vi "Example - Opening and Editing an Installer.vi"() -> ()   [LabVIEW 2017]
doc: "Demonstrates the use of the Installer Builder API to open, modify, and build an Installer build specification."
uses:
  <vilib>/InstallerBuilder/Classes/Win_Source/AB_Win_Source.lvclass/AB_Win_Source.ctl
  <vilib>/InstallerBuilder/Classes/Win_InstallTime_Executable/Install Time Type.ctl
  <vilib>/InstallerBuilder/Classes/Win_Installer/AB_Win_Installer.lvclass/AB_Win_Installer.ctl
  <vilib>/InstallerBuilder/Classes/Win_Source/Get Name.vi
  <vilib>/InstallerBuilder/Classes/Win_Source/Get Install Path.vi
  <vilib>/InstallerBuilder/Classes/Win_Installer/Get Product Name.vi
  <vilib>/InstallerBuilder/Classes/Win_Installer/Get Product Version.vi
  <vilib>/InstallerBuilder/Classes/Win_Source_File/AB_Win_Source_File.lvclass
  e:/builds/penguin/labview/branches/2017/dev/dist/vi.lib/InstallerBuilder/Classes/Win_Source/AB_Win_Source.lvclass
  <vilib>/InstallerBuilder/Classes/Win_Installer/Get Installed Files.vi
  <vilib>/InstallerBuilder/Classes/Win_Installer/Get System Folder (Desktop).vi
  <vilib>/InstallerBuilder/Classes/Win_Source_File/Set Read Only.vi
  <vilib>/InstallerBuilder/Classes/Win_Installer/Get Registry Hive (Local Machine).vi
  <vilib>/AppBuilder/AB_API_Simple/Build (project reference).vi
  <vilib>/InstallerBuilder/Classes/Win_Installer/AB_Win_Installer.lvclass
  <vilib>/AppBuilder/AB_API_Simple/NI_App_Builder_API.lvlib
  <vilib>/InstallerBuilder/Classes/Win_InstallTime_Executable/AB_Win_InstallTime_Executable.lvclass
panel:
  out "Files included in the installer":string[](array[string])
  # "Overview: Demonstrates the use of the Installer Builder API to open, modify, and build an Installer build specification.\nRequirements: LabVIEW Professional Development System or LabVIEW Application Builder\nInstructions:\n1. Run the VI. The My Installer build specification will be opened, modified, then built programmatically.\n2. A project window will open. Examine the My Installer build specification in the project.\n3. Close the temporary project and delete the temporary project files generated by this example when you are done.\n4. In the Project Explorer window, right-click on the My Installer build specification and choose Explore to navigate to the installer and run it."
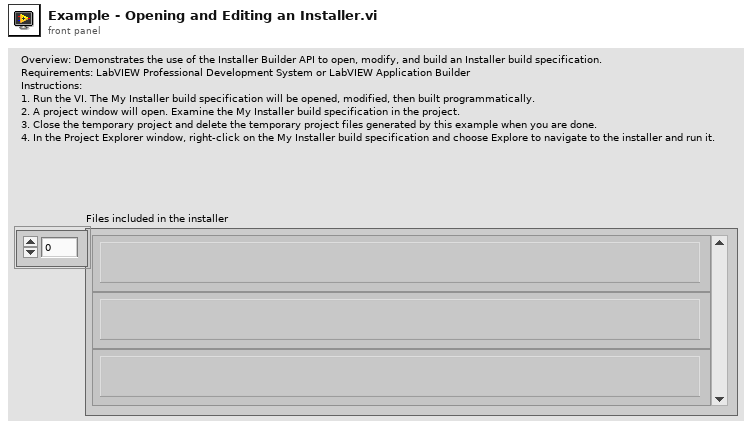
[diagram p1: front panel]
types:
  T1 = typedef "AB_Win_InstallTime_Executable.lvclass/Install Time Type.ctl" = enum16{"After install", "Before uninstall"}
  T2 = typedef "AB_Win_Installer.lvclass/Product Version.ctl" = cluster{"Major":u8, "Minor":u8, "Update":u16}
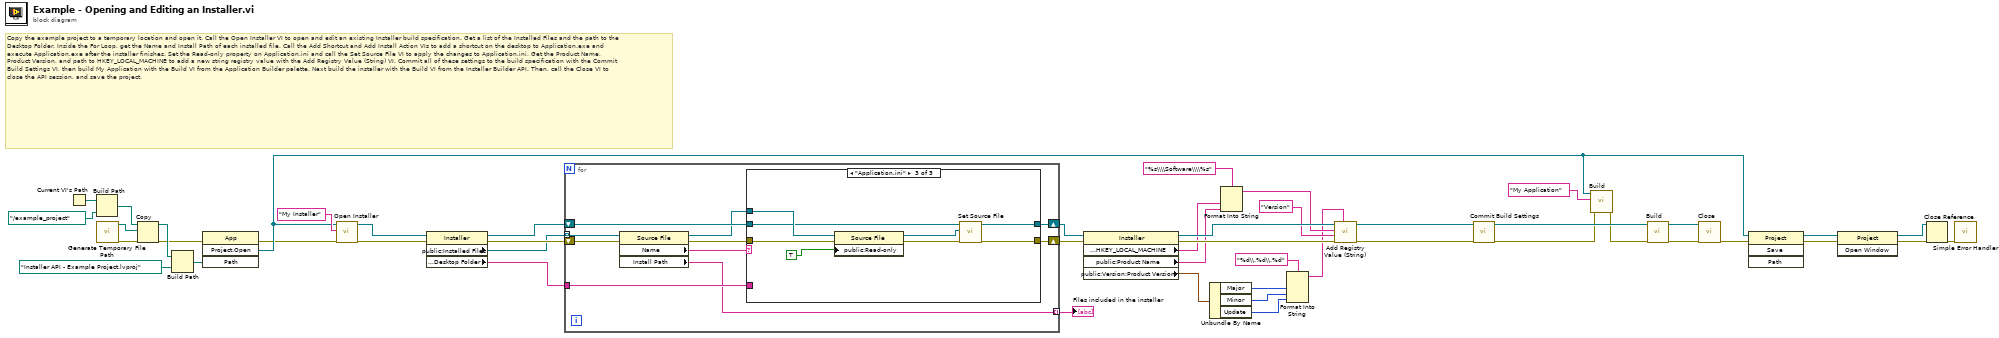
[diagram p0: block diagram]
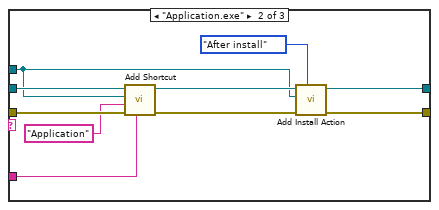
[diagram p3: hidden frame]
diagram:
  # "Copy the example project to a temporary location and open it. Call the Open Installer VI to open and edit an existing Installer build specification. Get a list of the Installed Files and the path to the Desktop Folder. Inside the For Loop, get the Name and Install Path of each installed file. Call the Add Shortcut and Add Install Action VIs to add a shortcut on the desktop to Application.exe and execute Application.exe after the installer finishes. Set the Read-only property on Application.ini and call the Set Source File VI to apply the changes to Application.ini. Get the Product Name, Product Version, and path to HKEY_LOCAL_MACHINE to add a new string registry value with the Add Registry Value (String) VI. Commit all of these settings to the build specification with the Commit Build Settings VI, then build My Application with the Build VI from the Application Builder palette. Next build the installer with the Build VI from the Installer Builder API. Then, call the Close VI to close the API session, and save the project."
  n1 = Current VI's Path() -> (path=w48:path)
  n2 = Build Path(base path=w48, name or relative path=path "../example_project" ("path")) -> (appended path=w46:path)
  n3 = call <vilib>:"Generate Temporary File Path.vi"() -> ("error out"=w40:errorcluster, "Unique Temporary File Path"=w45:path)  [unwired: 10 in]
  n4 = Copy(8:w40, 10:w45, 11:w46) -> (0:w39:errorcluster, 3:w44:path)  [unwired: 2 in, 1 out]
  n5 = Build Path(base path=w44, name or relative path=path "Installer API - Example Project.lvproj") -> (appended path=w42:path)
  n6 = invoke class="App" method="Project.Open"(error in=w39, "Path"=w42) -> (error out=w1:errorcluster, "Project:Open"=w6:refnum<vi>)  [unwired: 2 in, 2 out]
  n7 = call <vilib>:"Open Installer.vi"("error in (no error)"=w1, "Build Specification Name"="My Installer" ("Build specification name"), "Project Refnum"=w6) -> ("error out"=w29:errorcluster, "AB_Win_Installer out"=w37:refnum<class "AB_Win_Installer.lvclass">)  [unwired: 7 in]
  n8 = property class="Installer"(reference=w37, error in=w29) -> (reference out=w15:refnum<class "AB_Win_Installer.lvclass">, error out=w16:errorcluster, "public:Installed Files"=w14:refnum<class "AB_Win_Source_File.lvclass">[], "public:System Paths:Desktop Folder"=w13:string)
  n9 = for {
    tunnel: w14 -> [w58] mode=indexing
    shift-right: [w51] -> w33
    shift-left: w16 -> [w57]
    tunnel: [w49] -> w30 mode=indexing
    shift-right: [w55] -> w25
    shift-left: w15 -> [w56]
    tunnel: w13 -> [w53]
    n10 = property class="Source File"(reference=w58, error in=w57) -> (reference out=w54:refnum<class "AB_Win_Source_File.lvclass">, error out=w52:errorcluster, "Name"=w50:string, "Install Path"=w49:string)
    n11 = case shown="\"Application.ini\"" w50 {
      tunnel: w56 -> [w60 w70 w75]
      tunnel: [w60 w65 w74] -> w55
      tunnel: w54 -> [_ w61 w77]
      tunnel: w53 -> [_ w69 _]
      tunnel: w52 -> [w59 w68 w78]
      tunnel: [w59 w63 w73] -> w51
      frame Default {
      }
      frame "Application.exe" {
        n12 = call <vilib>:"Add Shortcut.vi"("Shortcut Path"=w69, "error in (no error)"=w68, "Shortcut Name"="Application", "Source File"=w61, "AB_Win_Installer in"=w70) -> ("error out"=w64:errorcluster, "AB_Win_Installer out"=w66:refnum<class "AB_Win_Installer.lvclass">)  [unwired: 4 in, 1 out]
        n13 = call <vilib>:"Add Install Action.vi"("Install Time Type"=Install_Time_Type."After install", "error in (no error)"=w64, "Source File"=w61, "AB_Win_Installer in"=w66) -> ("error out"=w63:errorcluster, "AB_Win_Installer out"=w65:refnum<class "AB_Win_Installer.lvclass">)  [unwired: 5 in, 1 out]
      }
      frame "Application.ini" {
        n14 = property class="Source File"(reference=w77, error in=w78, "public:Read-only"=TRUE ("Read-only")) -> (reference out=w71:refnum<class "AB_Win_Source_File.lvclass">, error out=w72:errorcluster)
        n15 = call <vilib>:"Set Source File.vi"("error in (no error)"=w72, "Source File"=w71, "AB_Win_Installer in"=w75) -> ("error out"=w73:errorcluster, "AB_Win_Installer out"=w74:refnum<class "AB_Win_Installer.lvclass">)  [unwired: 7 in]
      }
    }
  }
  "Files included in the installer" <- w30
  n16 = property class="Installer"(reference=w25, error in=w33) -> (reference out=w24:refnum<class "AB_Win_Installer.lvclass">, error out=w23:errorcluster, "public:Registry Hives:HKEY_LOCAL_MACHINE"=w19:string, "public:Product Name"=w18:string, "public:Version:Product Version"=w12:T2)
  n17 = Unbundle By Name(w12) -> ("Major"=w10:u8, "Minor"=w9:u8, "Update"=w8:u16)
  n18 = Format Into String(format string="%s\\\\Software\\\\%s", w19, w18) -> (resulting string=w17:string)  [unwired: 2 in, 1 out]
  n19 = Format Into String(format string="%d\\.%d\\.%d", w10, w9, w8) -> (resulting string=w7:string)  [unwired: 2 in, 1 out]
  n20 = call <vilib>:"Add Registry Value (String).vi"("Value Data"=w7, "error in (no error)"=w23, "Value Name"="Version" ("Key"), "Key"=w17, "AB_Win_Installer in"=w24) -> ("error out"=w22:errorcluster, "AB_Win_Installer out"=w26:refnum<class "AB_Win_Installer.lvclass">)  [unwired: 4 in, 1 out]
  n21 = call <vilib>:"Commit Build Settings.vi"("error in (no error)"=w22, "AB_Win_Installer in"=w26) -> ("error out"=w32:errorcluster, "AB_Win_Installer out"=w34:refnum<class "AB_Win_Installer.lvclass">)  [unwired: 8 in]
  n22 = call-poly <vilib>:"Build.vi"("error in (no error)"=w32, "Name of build specification (if empty: build all)"="My Application" ("Name"), "Project reference"=w6) -> ("error out"=w31:errorcluster)  [unwired: 6 in, 2 out]
  n23 = call <vilib>:"Build.vi"("error in (no error)"=w31, "AB_Win_Installer in"=w34) -> ("error out"=w35:errorcluster, "AB_Win_Installer out"=w36:refnum<class "AB_Win_Installer.lvclass">)  [unwired: 8 in]
  n24 = call <vilib>:"Close.vi"("error in (no error)"=w35, "AB_Win_Installer in"=w36) -> ("error out"=w28:errorcluster)  [unwired: 9 in]
  n25 = invoke class="Project" method="Save"(reference=w6, error in=w28) -> (reference out=w5:refnum<vi>, error out=w3:errorcluster)  [unwired: 2 in, 2 out]
  n26 = invoke class="Project" method="Open Window"(reference=w5, error in=w3) -> (reference out=w4:refnum<vi>, error out=w2:errorcluster)  [unwired: 1 in, 1 out]
  n27 = Close Reference(reference=w4, error in (no error)=w2) -> (error out=w47:errorcluster)
  n28 = call <vilib>:"Simple Error Handler.vi"("error in (no error)"=w47) -> ()  [unwired: 4 in, 5 out]
